vi "AttrMap-SetValue2.vi"(8 "error in (no error)":errorcluster, 9 "Key":string, 10 "Value":variant, 11 "AttrMap in":T1) -> (0 "error out":errorcluster, 3 "AttrMap out":T1)   [LabVIEW 2019, in "lv-apt-json-file.lvlib"]
uses:
  lv-apt-json-file.lvlib
  Typedef/Def-AttrMap.ctl
  6e91e2cf-a420-477d-bf86-627245081caf.vi
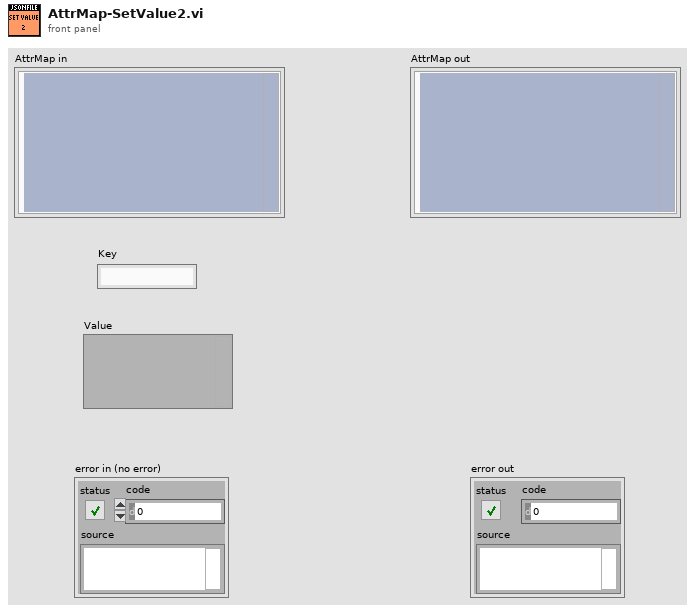
[diagram p1: front panel]
types:
  T1 = typedef "lv-apt-json-file.lvlib/Def-AttrMap.ctl" = cluster{"Map":variant}
  T2 = typedef "lv-apt-json-file.lvlib/Def-NameMap.ctl" = variant[]
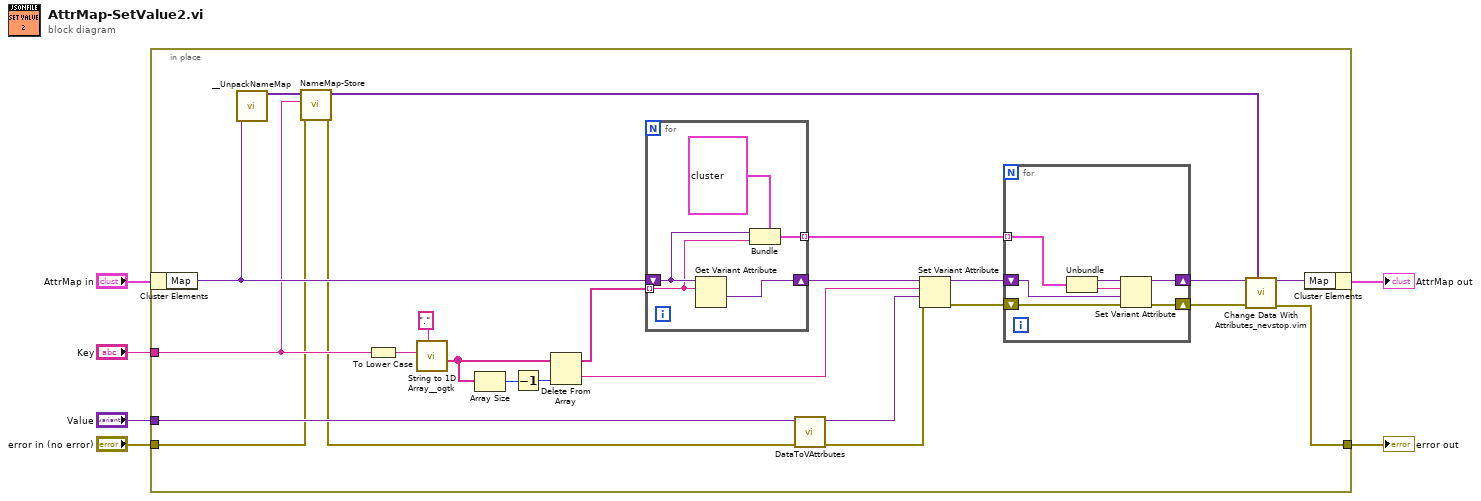
[diagram p0: block diagram]
diagram:
  n1 = in-place {
    in-place-border: [w30] -> w6
    in-place-border: "error in (no error)" -> [w10]
    in-place-border: "Key" -> [w11]
    in-place-border: "Value" -> [w16]
    n2 = in-place-cluster #1("AttrMap in") -> ("Map"=w27:variant)
    n3 = call "__UnpackNameMap.vi"("Map"=w27) -> ("NameMap"=w13:T2)  [unwired: 10 in]
    n4 = call "NameMap-Store.vi"("error in (no error)"=w10, "name"=w11, "NameMap in"=w13) -> ("error out"=w9:errorcluster, "NameMap out"=w12:T2)  [unwired: 7 in]
    n5 = To Lower Case(string=w11) -> (all lower case string=w25:string)
    n6 = call <userlib>:"String to 1D Array__ogtk.vi"("delimiter (Tab)"=".", "string"=w25) -> ("Array of Strings"=w22:string[])  [unwired: 9 in]
    n7 = Array Size(array=w22) -> (size(s)=w26:i32)
    n8 = Decrement(x=w26) -> (x-1=w17:i32)
    n9 = Delete From Array(array=w22, index=w17) -> (deleted portion=w23:string, array with subset deleted=w21:string[])  [unwired: 1 in]
    n10 = for {
      tunnel: w21 -> [w41] mode=indexing
      shift-right: [w40] -> w24
      shift-left: w27 -> [w42]
      tunnel: [w38] -> w20 mode=indexing
      n11 = Get Variant Attribute(Variant=w42, name=w41) -> (value=w40:variant)  [unwired: 2 in, 3 out]
      n12 = Bundle(cluster=cluster{"Parent":variant, "Name":string} {"Parent"=variant, "Name"=""}, "Parent"=w42, "Name"=w41) -> (w38:cluster{"Parent":variant, "Name":string})
    }
    n13 = call "DataToVAttrbutes.vi"("error in (no error)"=w9, "data"=w16) -> ("error out"=w14:errorcluster, "VAttributes"=w15:variant)  [unwired: 8 in]
    n14 = Set Variant Attribute(Variant=w24, name=w23, value=w15, error in=w14) -> (Variant out=w19:variant, error out=w8:errorcluster)  [unwired: 1 out]
    n15 = for {
      tunnel: w20 -> [w37] mode=indexing
      shift-right: [w36] -> w18
      shift-left: w19 -> [w33]
      shift-right: [w31] -> w7
      shift-left: w8 -> [w32]
      n16 = Unbundle(w37) -> ("Parent"=w35:variant, "Name"=w34:string)
      n17 = Set Variant Attribute(Variant=w35, name=w34, value=w33, error in=w32) -> (Variant out=w36:variant, error out=w31:errorcluster)  [unwired: 1 out]
    }
    n18 = call "Change Data With Attributes_nevstop.vim"("Data"=w12, "error in (no error)"=w7, "Variant in"=w18) -> ("error out"=w30:errorcluster, "Variant out"=w29:variant)  [unwired: 7 in]
    n19 = in-place-cluster #1("Map"=w29) -> (→"AttrMap out":T1)
  }
  "error out" <- w6
